vi "Create Camera Process.vi"(8 "error in (no error)":errorcluster, 10 "Camera Driver.lvclass":refnum<class "Camera Driver.lvclass">, 11 "Camera Controller in":refnum<class "Camera Controller.lvclass">) -> (0 "error out":errorcluster, 3 "Camera Controller":refnum<class "Camera Controller.lvclass">)   [LabVIEW 2022 SP3, in "Cam Process.lvlib" / "Camera Process.lvclass"]
uses:
  Camera Process.lvclass
  Camera Controller/Camera Controller.lvclass
  Camera Driver/Camera Driver.lvclass
  C:/Program Files/National Instruments/LabVIEW 2022/vi.lib/ActorFramework/Actor/Actor.lvclass
  Camera Process.lvclass/Camera Process.ctl
  XY Stage/Process Actor/Process Framework/Process State Data/Process State Data.lvclass
  XY Stage/Process Actor/Process Framework/Interlock Q Class/Interlock Q Class.lvclass
  <vilib>/ActorFramework/Actor/Actor.lvclass
  Camera Data/Camera Data.lvclass
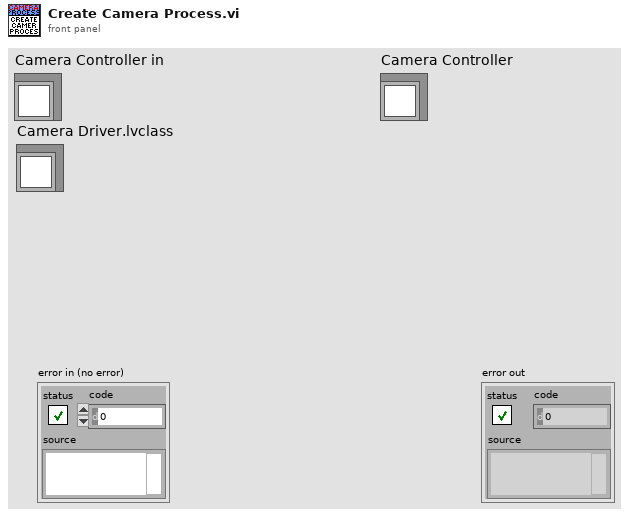
[diagram p1: front panel]
types:
  T1 = typedef "Image Type" = u32
  T2 = typedef "IMAQ Image.ctl" = refnum<image>
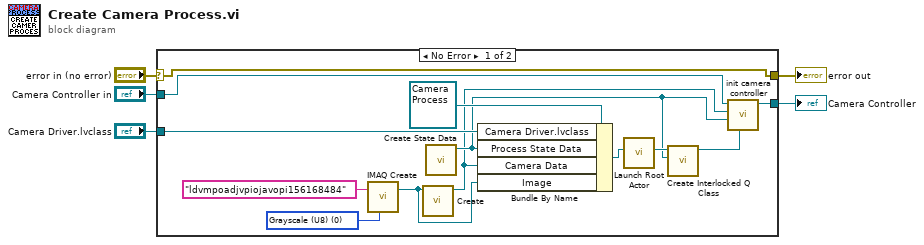
[diagram p0: block diagram]
diagram:
  n1 = case shown="No Error" "error in (no error)" {
    selector: "error in (no error)" -> [w18 w20]
    tunnel: [w18 w20] -> w4
    tunnel: "Camera Driver.lvclass" -> [w16 _]
    tunnel: "Camera Controller in" -> [w11 w19]
    tunnel: [w8 w19] -> w1
    frame No Error {
      w6 = T1 0 items=["Grayscale (U8)", "Grayscale (I16)", "Grayscale (SGL)", "Complex (CSG)", "RGB (U32)", "HSL (U32)", "RGB (U64)", "Grayscale (U16)"] ("Image Type")
      n2 = call "IMAQ Create"("Image Name"="ldvmpoadjvpiojavopi156168484", "Image Type"=w6) -> ("New Image"=w7:T2)  [unwired: 3 in, 1 out]
      n3 = call "Create.vi"("Image"=w7) -> ("Camera Data"=w10:refnum<data-value>)  [unwired: 9 in, 1 out]
      n4 = call "Create State Data.vi"() -> ("Process State Data out"=w12:refnum<data-value>)  [unwired: 10 in, 1 out]
      n5 = Bundle By Name(cluster=refnum<class "Camera Process.lvclass"> refnum ("Camera Process.lvclass"), "Camera Driver.lvclass"=w16, "Process State Data"=w12, "Camera Data"=w10, "Image"=w7) -> (w15:refnum<class "Camera Process.lvclass">)
      n6 = call <vilib>:"Launch Root Actor.vi"("Actor"=w15) -> ("Actor's Enqueuer"=w14:refnum<class "Message Enqueuer.lvclass">)  [unwired: 9 in, 1 out]
      n7 = call "Create Interlocked Q Class.vi"("Process State Data"=w12, "Process Q"=w14) -> ("Interlock Q Class out"=w13:refnum<class "Interlock Q Class.lvclass">)  [unwired: 9 in]
      n8 = call "init camera controller.vi"("Interlock Q Class out"=w13, "Process State Data out"=w12, "Camera Data"=w10, "Camera Controller in"=w11) -> ("Camera Controller out"=w8:refnum<class "Camera Controller.lvclass">)  [unwired: 6 in, 1 out]
    }
    frame Error {
    }
  }
  "error out" <- w4
  "Camera Controller" <- w1
